vi "RSZVB Marker Search Results.vi"(8 "error in (no error)":errorcluster {"code" format="%.0x"}, 9 "Marker (1)":i32=1, 10 "Channel (Trace) (1)":i32=1, 11 "VISA session":refnum<visa-resource-name>) -> (0 "error out":errorcluster {"code" format="%.0x"}, 1 "Marker Response":dbl[](array[numeric]) format="%^.3e", 2 "Marker Stimulus":dbl format="%^.3e", 3 "dup VISA session":refnum<visa-resource-name>)   [LabVIEW 2011]
doc: "This VI Returns the result (stimulus and response value) of a search started by means of CALCulate<Ch/Tr>:MARKer<Mk>:FUNCtion:EXECute. The search must be executed before the command is enabled.\n\nRemote-control command(s):\nCALCulate<Ch/Tr>:MARKer<Mk>:FUNCtion:RESult?"
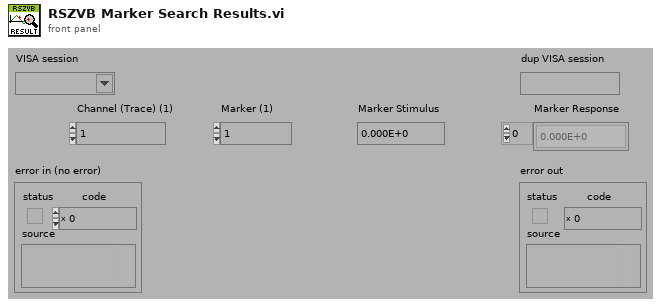
[diagram p1: front panel]
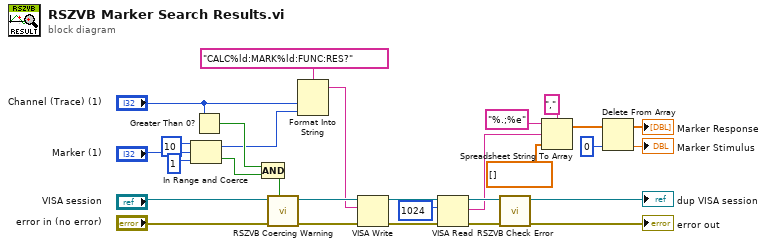
[diagram p0: block diagram]
diagram:
  n1 = In Range and Coerce(upper limit=10, x="Marker (1)", lower limit=1) -> (coerced(x)=w20:i32, In Range?=w23:bool)
  n2 = Greater Than 0?(x="Channel (Trace) (1)") -> (x > 0?=w26:bool)
  n3 = Compound Arithmetic op=AND(w26, w23) -> (w22:bool)
  n4 = call "RSZVB Coercing Warning.vi"("In Range?"=w22, "error in (no error)"="error in (no error)", "VISA session"="VISA session") -> ("error out"=w28:errorcluster, "dup VISA session"=w29:refnum<visa-resource-name>)  [unwired: 7 in]
  n5 = Format Into String(format string="CALC%ld:MARK%ld:FUNC:RES?", "Channel (Trace) (1)", w20) -> (resulting string=w21:string)  [unwired: 2 in, 1 out]
  n6 = VISA Write(VISA resource name=w29, write buffer=w21, error in (no error)=w28) -> (VISA resource name out=w14:refnum<visa-resource-name>, error out=w13:errorcluster)  [unwired: 1 out]
  n7 = VISA Read(VISA resource name=w14, byte count=u32 1024 ("byte count (0)"), error in (no error)=w13) -> (VISA resource name out=w16:refnum<visa-resource-name>, read buffer=w1:string, error out=w15:errorcluster)  [unwired: 1 out]
  n8 = call "RSZVB Check Error.vi"("error in (no error)"=w15, "VISA session"=w16) -> ("error out"=→"error out":errorcluster, "dup VISA session"=→"dup VISA session":refnum<visa-resource-name>)  [unwired: 8 in]
  n9 = Spreadsheet String To Array(delimiter (Tab)=",", format string="%.;%e", spreadsheet string=w1, array type (2D Dbl)=dbl[] []) -> (array=w6:dbl[])
  n10 = Delete From Array(array=w6, index=0) -> (deleted portion=→"Marker Stimulus":dbl, array with subset deleted=→"Marker Response":dbl[])  [unwired: 1 in]
